vi "Get Enable State.vi"(8 "error in (no error)":errorcluster, 11 "Abs_Value.lvclass in":refnum<class "Abs_Value.lvclass">) -> (0 "error out":errorcluster, 2 "Enabled?":bool, 3 "Abs_Value.lvclass out":refnum<class "Abs_Value.lvclass">)   [LabVIEW 2021, in "Fault-Injection_Type.lvclass"]
uses:
  <vilib>/TSA/Abstract Data Classes/Abs_Types/Value/Abs_Value.lvclass
  Support/Interfaces/Type/Fault-Injection_Type.lvclass
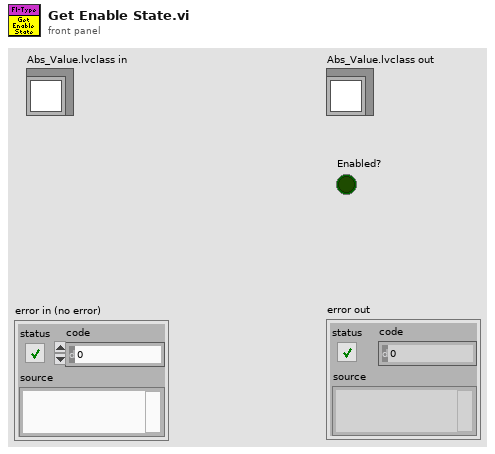
[diagram p1: front panel]
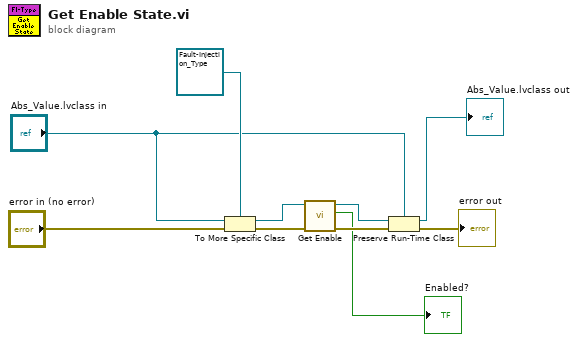
[diagram p0: block diagram]
diagram:
  n1 = To More Specific Class(target class=refnum<class "Fault-Injection_Type.lvclass"> refnum ("Fault-Injection_Type.lvclass"), reference="Abs_Value.lvclass in", error in="error in (no error)") -> (specific class reference=w5:refnum<class "Fault-Injection_Type.lvclass">, error out=w2:errorcluster)
  n2 = call-dynamic "Get Enable.vi"("error in (no error)"=w2, "Fault-Injection_Type in"=w5) -> ("error out"=w3:errorcluster, "Enable?"=→"Enabled?":bool, "Fault-Injection_Type out"=w4:refnum<class "Fault-Injection_Type.lvclass">)  [unwired: 7 in]
  n3 = Preserve Run-Time Class(object in=w4, error in=w3, 2:"Abs_Value.lvclass in") -> (object out=→"Abs_Value.lvclass out":refnum<class "Abs_Value.lvclass">, error out=→"error out":errorcluster)
